vi "get label.vi"(8 "error in (no error)":errorcluster caption="Fehler (Eingang, kein Fehler)", 11 "img (Eingang)":refnum<class "img.lvclass">) -> (0 "error out":errorcluster caption="Fehler (Ausgang)", 2 "label":string, 3 "img (Ausgang)":refnum<class "img.lvclass">)   [LabVIEW 2013, in "DatenKlassen.lvlib" / "img.lvclass"]
uses:
  img.lvclass
  img.lvclass/img.ctl
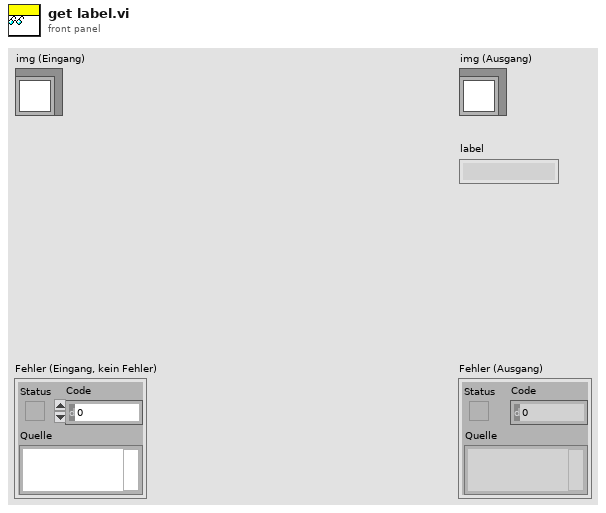
[diagram p1: front panel]
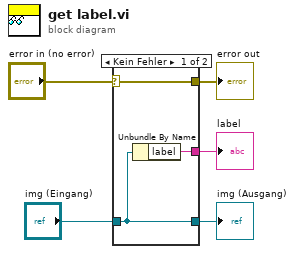
[diagram p0: block diagram]
diagram:
  n1 = case shown="Kein Fehler" "error in (no error)" {
    selector: "error in (no error)" -> [w8 w9]
    tunnel: [w8 w9] -> w4
    tunnel: [w7 w10] -> w2
    tunnel: "img (Eingang)" -> [w7 w10]
    tunnel: [w6 _] -> w1
    frame No Error {
      n2 = Unbundle By Name(w7) -> ("label"=w6:string)
    }
    frame Error {
    }
  }
  "error out" <- w4
  "img (Ausgang)" <- w2
  "label" <- w1
